vi "APSxSensorBitsToString.vi"(8 "error in (no error)":errorcluster caption="错误输入（无错误）", 9 "BufferSize":i32, 10 "InitialBitString in":string, 11 "hSENSOR":i32) -> (0 "error out":errorcluster caption="错误输出", 1 "Message":string, 2 "InitialBitString":string, 3 "hSENSOR out":i32)   [LabVIEW 2018]
doc: "该模板用于创建子VI。"
uses:
  APSx.dll/APSx.dll
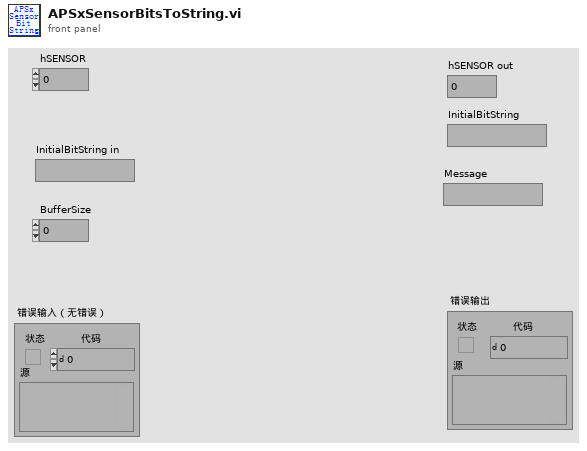
[diagram p1: front panel]
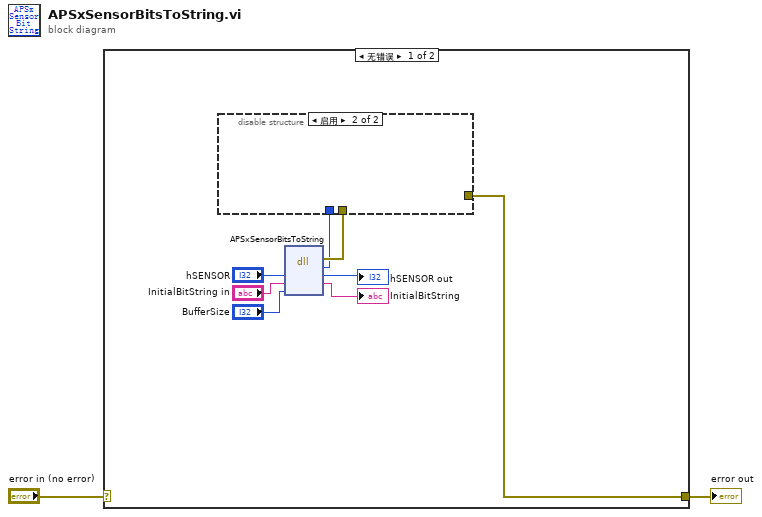
[diagram p0: block diagram]
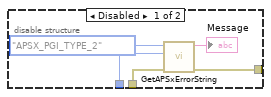
[diagram p2: hidden frame]
diagram:
  n1 = case shown="无错误" "error in (no error)" {
    selector: "error in (no error)" -> [_ w16]
    tunnel: [w10 w16] -> w1
    frame No Error {
      n2 = dll-call lib="PTH2]abs D项目Feng恒隆项目Labview传感器对中台SourcesAPSx.dllAPSx.dll" fn="APSxSensorBitsToString"("hSENSOR"="hSENSOR", "Buffer"="InitialBitString in", "BufferSize"="BufferSize") -> (error out=w4:errorcluster, "Code"=w3:i32, "hSENSOR"=→"hSENSOR out":i32, "Buffer"=→"InitialBitString":string)  [unwired: 4 in, 1 out]
      n3 = disable-structure shown="启用" {
        disable-tunnel: w4 -> [w15 _]
        disable-tunnel: w3 -> [w14 _]
        disable-tunnel: [w12 _] -> w10
        frame Disabled {
          n4 = call "GetAPSxErrorString.vi"("error in (no error)"=w15, "ErrorCode"=w14, "PGIType"=enum16{"APSX_PGI_TYPE_1", "APSX_PGI_TYPE_2"}."APSX_PGI_TYPE_2") -> ("error out"=w12:errorcluster, "Message"=→"Message":string)  [unwired: 7 in]
        }
        frame Enabled {
        }
      }
    }
    frame Error {
    }
  }
  "error out" <- w1
